vi "Resolve Resource.vi"(6 "headers in":T1[](array[typedef]), 7 "Parameters":string[](array[string]), 8 "error in (no error)":errorcluster, 9 "Method name":string, 10 "Resource name":string, 11 "RESTful Service in":refnum<class "REST Client.lvclass">) -> (0 "error out":errorcluster, 1 "Resolved method":T2, 2 "Resolved URL":string, 3 "RESTful Service out":refnum<class "REST Client.lvclass">, 4 "headers out":T1[](array[typedef]))   [LabVIEW 2013]
uses:
  Resource/Resource.lvclass
  REST Client.lvclass
  <vilib>/wsapi/NI_WebServices.lvlib
  HTTP Methods.ctl
  HTTP Header.ctl
panel:
  # "Copyright © 2014 JKI All rights reserved.\n\nAuthor: Tomi Maila <tomi.maila@jki.net>\n\nThis library is provided \"AS IS\" ,WITHOUT WARRANTIES OR \nCONDITIONS OF ANY KIND, either express or implied.\n\nJKI -- jki.net"
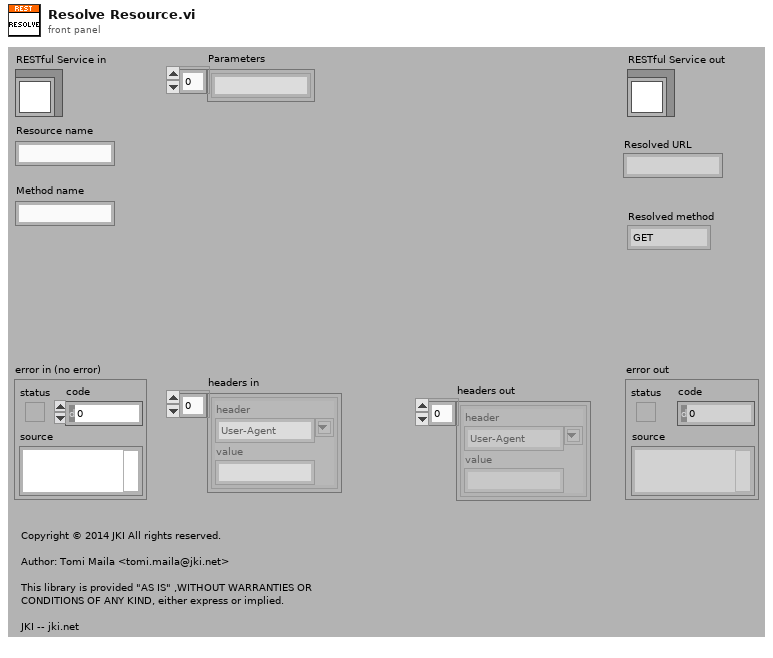
[diagram p1: front panel]
types:
  T1 = typedef "REST Client.lvclass/HTTP Header.ctl" = cluster{"header":string, "value":string}
  T2 = typedef "REST Client.lvclass/HTTP Methods.ctl" = enum16{"GET", "HEAD", "POST", "PUT", "DELETE"}
  T3 = typedef "Resource Method.ctl" = cluster{"Name":string, "HTTP method":T2, "Append trailing slash":bool, "Remove trailing slash":bool, "Parameters":string[]}
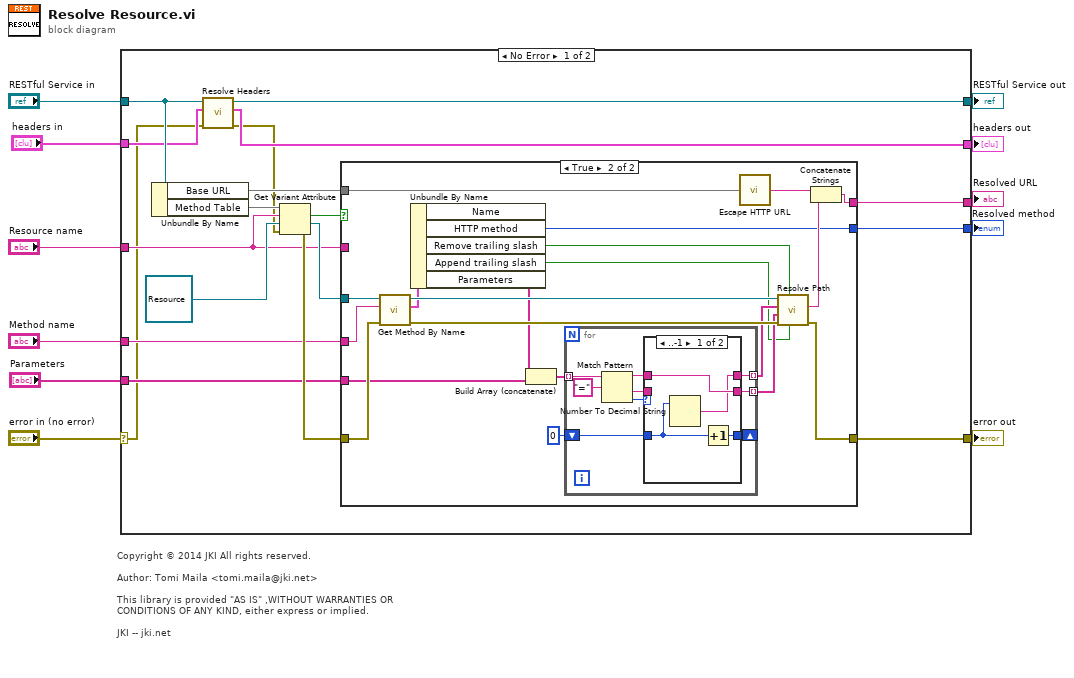
[diagram p0: block diagram]
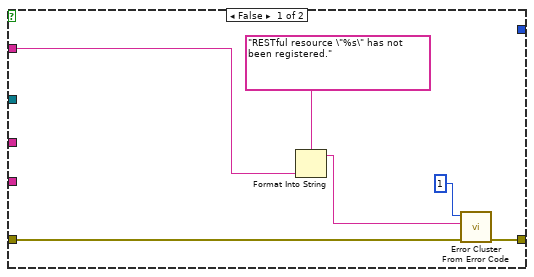
[diagram p2: hidden frame]
diagram:
  # "Copyright © 2014 JKI All rights reserved.\n\nAuthor: Tomi Maila <tomi.maila@jki.net>\n\nThis library is provided \"AS IS\" ,WITHOUT WARRANTIES OR \nCONDITIONS OF ANY KIND, either express or implied.\n\nJKI -- jki.net"
  n1 = case shown="No Error" "error in (no error)" {
    selector: "error in (no error)" -> [w13 w73]
    tunnel: [w24 w73] -> w10
    tunnel: [w17 w72] -> w8
    tunnel: "RESTful Service in" -> [w18 w72]
    tunnel: "Resource name" -> [w23 _]
    tunnel: "Method name" -> [w22 _]
    tunnel: "Parameters" -> [w21 _]
    tunnel: [w12 _] -> w4
    tunnel: [w19 _] -> w3
    tunnel: [w15 _] -> w2
    tunnel: "headers in" -> [w16 _]
    frame No Error {
      n2 = Unbundle By Name(w18) -> ("Base URL"=w20, "Method Table"=w29)
      n3 = call "Resolve Headers.vi"("error in (no error)"=w13, "headers in"=w16, "REST Client in"=w18) -> ("error out"=w14:errorcluster, "headers out"=w15:T1[], "REST Client out"=w17:refnum<class "REST Client.lvclass">)  [unwired: 6 in]
      n4 = Get Variant Attribute(Variant=w29, name=w23, default value (empty Variant)=refnum<class "Resource.lvclass"> refnum ("Resource.lvclass"), error in=w14) -> (found=w27:bool, value=w26:refnum<class "Resource.lvclass">, error out=w25:errorcluster)  [unwired: 1 out]
      n5 = case shown="True" w27 {
        tunnel: w26 -> [_ w55]
        tunnel: w25 -> [w35 w53]
        tunnel: [w34 w42] -> w24
        tunnel: w23 -> [w31 _]
        tunnel: w22 -> [_ w54]
        tunnel: w21 -> [_ w39]
        tunnel: w20 -> [_ w36]
        tunnel: [_ w44] -> w12
        tunnel: [_ w43] -> w19
        frame False {
          n6 = Format Into String(format string="RESTful resource \"%s\" has not been registered." ("error message (\"\")"), w31) -> (resulting string=w30:string)  [unwired: 2 in, 1 out]
          n7 = call <vilib>:"Error Cluster From Error Code.vi"("error in (no error)"=w35, "error message (\"\")"=w30, "error code (0)"=1) -> ("error out"=w34:errorcluster)  [unwired: 6 in]
        }
        frame True {
          n8 = call-dynamic "Get Method By Name.vi"("error in (no error)"=w53, "Name"=w54, "Resource in"=w55) -> ("error out"=w51:errorcluster, "Method"=w48:T3, "Resource out"=w52:refnum<class "Resource.lvclass">)  [unwired: 6 in]
          n9 = Unbundle By Name(w48) -> ("HTTP method"=w43:T2, "Remove trailing slash"=w47:bool, "Append trailing slash"=w46:bool, "Parameters"=w40:string[])  [unwired: 1 out]
          n10 = Build Array (concatenate)(w40, w39) -> (w41:string[])
          n11 = for {
            tunnel: w41 -> [w64] mode=indexing
            tunnel: [w58] -> w50 mode=indexing
            tunnel: [w59] -> w49 mode=indexing
            shift-right: [w56] -> _
            shift-left: 0 -> [w57]
            n12 = Match Pattern(string=w64, regular expression="=") -> (before substring=w61:string, after substring=w60:string, offset past match=w63:i32)  [unwired: 1 in, 1 out]
            n13 = case shown="..-1" w63 {
              tunnel: w61 -> [w68 w70]
              tunnel: w60 -> [_ w71]
              tunnel: [w68 w71] -> w59
              tunnel: [w65 w70] -> w58
              tunnel: w57 -> [w66 w69]
              tunnel: [w67 w69] -> w56
              frame ..-1 {
                n14 = Number To Decimal String(number=w66) -> (decimal integer string=w65:string)  [unwired: 1 in]
                n15 = Increment(x=w66) -> (x+1=w67:i32)
              }
              frame 0.. {
              }
            }
          }
          n16 = call <vilib>:"Escape HTTP URL.vi"("unescaped string in"=w36) -> ("escaped string out"=w37:string)
          n17 = call-dynamic "Resolve Path.vi"("Append trailing slash (F)"=w46, "Remove trailing slash (F)"=w47, "error in (no error)"=w51, "Values in"=w49, "Keys in"=w50, "Resource in"=w52) -> ("error out"=w42:errorcluster, "Path"=w45:string)  [unwired: 3 in, 1 out]
          n18 = Concatenate Strings(w37, w45) -> (w44:string)
        }
      }
    }
    frame Error {
    }
  }
  "error out" <- w10
  "RESTful Service out" <- w8
  "Resolved URL" <- w4
  "Resolved method" <- w3
  "headers out" <- w2
